vi "Teleop.vi"(10 "Match Info":T4={"Autonomous Elapsed Seconds"=0.0, "TeleOp Elapsed Seconds"=0.0, "Disabled Elapsed Seconds"=0.0, "Visited Autonomous"=FALSE, "Visited TeleOp"=FALSE, "Visited Disabled"=FALSE, "Autonomous Settings"={"Autonomous Style"=enum."Independent", "VI Refnum"=refnum}}, 11 "Call Context":T5) -> ()   [LabVIEW 2018]
doc: "This VI is called for each TeleOp packet received from the DS where the robot is not disabled. It is often used to read from the joysticks and update I/O or to update setpoints for timed control loops. It should complete and return within 20 milliseconds or it may miss DS packets."
uses:
  <vilib>/Rock Robotics/WPI/DriverStation/WPI_DriverStationDerivedRobotMode.ctl
  <vilib>/Rock Robotics/WPI/DriverStation/WPI_DriverStationMatch Info.ctl
  <vilib>/Rock Robotics/WPI/Solenoid/WPI_SolenoidValue.ctl
  <vilib>/Rock Robotics/WPI/ThirdParty/Phoenix-LabVIEW/Motor Controller/Controls/CTRE_Phoenix_MotorControl_ControlMode.ctl
  <vilib>/Rock Robotics/WPI/Utilities/WPI_GetSetVariantRefNum.vi
  <vilib>/Rock Robotics/WPI/Joystick/WPI_JoystickArcadeMapping.vi
  <vilib>/Rock Robotics/Network Tables/NT Write Boolean Array.vi
  <vilib>/Rock Robotics/Network Tables/NT Write Numeric Array.vi
  <vilib>/Rock Robotics/WPI/Solenoid/WPI_SolenoidSetEnum.vi
  <vilib>/Rock Robotics/WPI/ThirdParty/Phoenix-LabVIEW/Motor Controller/Get/CTRE_Phoenix_MotorController_GetSelectedSensorData.vi
  <vilib>/Rock Robotics/Network Tables/NT Read Boolean.vi
  Toolbox/Simple Limit Switch/Limits(Switch+Encoder).vi
  Toolbox/Simple Limit Switch/Limits(DoubleSwitch).vi
  Toolbox/Simple Limit Switch/Limits(SingleSwitch).vi
  <vilib>/Rock Robotics/Network Tables/NT Write Number.vi
panel:
  out "Wrist  Encoder Value":i32
  out "Wrist Out":dbl
  out "Wrist PID Out":dbl
  out "Elevator Out":dbl
  out "Elevator PID Out":dbl
  in  "Outer Invert Motor Limit":bool
  in  "Outer Invert Encoder Limit":bool=TRUE
  in  "Outer Limit":dbl format="%#_13g"
  in  "Horse Invert Encoder Limit":bool=TRUE
  in  "Wrist Invert Encoder Limit":bool=TRUE
  in  "Elevator Invert Encoder Limit":bool=TRUE
  out "Horse Limit Switch":bool
  in  "Reset Horse Encoder":bool
  out "OuterStageSwitch":bool
  out "Wrist After Dangerzone":T1(ring)
  out "Elevator  After Dangerzone":T2(ring)
  in  "Elevator Auto":bool=TRUE
  in  "Elevator Output Range":cluster{"output high":dbl, "output low":dbl}={"output high"=0.2, "output low"=-0.75}
  in  "Elevator PID Gains":T3={"proportional gain (Kc)"=-1e-05, "integral time (Ti, min)"=0.0, "derivative time (Td, min)"=0.0}
  in  "Elevator Setpoints":dbl[](array[numeric])=[-10000.0, -10000.0, -10000.0, 267000.0, 237000.0, 440000.0]
  in  "Wrist Auto":bool=TRUE
  in  "Wrist Output Range":cluster{"output high":dbl, "output low":dbl}={"output high"=0.5, "output low"=-0.5}
  in  "Wrist PID Gains":T3={"proportional gain (Kc)"=2e-05, "integral time (Ti, min)"=0.0, "derivative time (Td, min)"=0.0}
  in  "Wrist Invert Motor Limit":bool=TRUE
  out "Wrist Limit Switch":bool
  out "Elevator Limit Switch Top":bool
  in  "Elevator Invert Motor Limit":bool=TRUE
  in  "Intake Encoder Limit":dbl=-130000.0 format="%#_13g"
  in  "Intake Home Encoder Limit":dbl=-45000.0 format="%#_13g"
  in  "HorseDanger":i32=-600000
  in  "Horse  Encoder Limit":dbl=-190000.0 format="%#_13g"
  in  "Horse Invert Motor Limit":bool=TRUE
  out "Elevator Limit Switch":bool
  out "Elevator Encoder":i32=-47
  in  "Reset Elevator Encoder":bool
  out "Horse Encoder":i32
  in  "Reset Wrist Encoder":bool
  out "Intake Wrist Encoder":i32
  # "BETA POWER/DIRECTIONS\nElevator: Negative is up\nHorse: Negative is into robot\nOuter: Positive is down\nWrist: Negative is into robot"
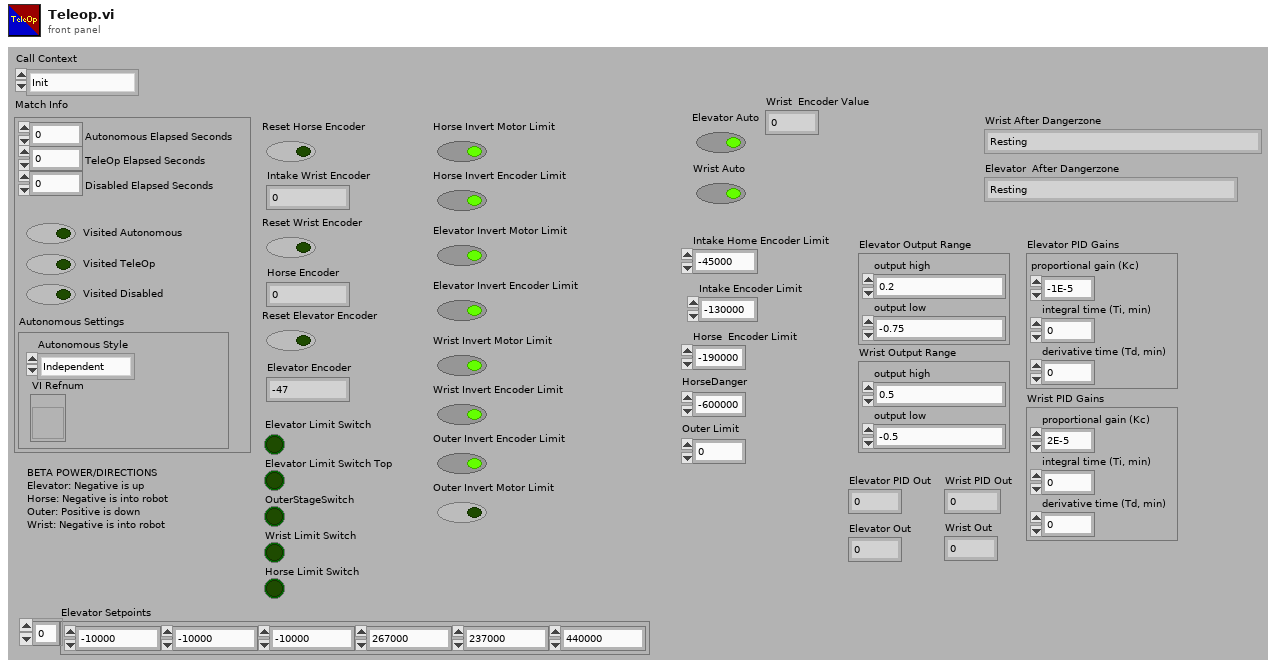
[diagram p1: front panel]
types:
  T1 = enum16{"Resting", "Hatch Ground Intake", "Hatch Place Low/Mid/CargoShip", "Hatch Place High", "Cargo Ground Intake", "Cargo Place Low/Mid", "Cargo Place High", "CargoShip Place Front", "CargoShip Place Back"}
  T2 = enum16{"Resting", "CargoShip Front", "CargoShip Back", "Cargo Mid", "Hatch Mid", "All High"}
  T3 = cluster{"proportional gain (Kc)":dbl, "integral time (Ti, min)":dbl, "derivative time (Td, min)":dbl}
  T4 = typedef "WPI_DriverStationMatch Info.ctl" = cluster{"Autonomous Elapsed Seconds":dbl, "TeleOp Elapsed Seconds":dbl, "Disabled Elapsed Seconds":dbl, "Visited Autonomous":bool, "Visited TeleOp":bool, "Visited Disabled":bool, "Autonomous Settings":cluster{"Autonomous Style":enum16{"Iterative", "Independent"}, "VI Refnum":refnum<vi>}}
  T5 = typedef "WPI_DriverStationDerivedRobotMode.ctl" = enum16{"Init", "Execute", "Stop"}
  T6 = typedef "WPI_SolenoidValue.ctl" = enum16{"Off", "On", "Forward", "Reverse"}
  T7 = enum16{"Intake Cargo", "Outtake Cargo", "Resting Cargo", "Intake Hatches", "Outtake Hatches", "Resting Hatches"}
  T8 = enum16{"Elevator Level 1", "Elevator Level 2", "Elevator Level 3"}
  T9 = typedef "CTRE_Phoenix_MotorControl_ControlMode.ctl" = u16
  T10 = cluster{"Intake Wheels Forwards":bool, "Elevator Shift":bool, "Intake Wheels Backwards":bool, "Drivetrain Shift":bool, "Elevator Outer Forwards":bool, "Elevator Outer Backwards":bool, "Hatch Telescope":bool, "Hatch Intake Clamp":bool, "Horse Drive Up":bool, "Horse Drive Down":bool, "Level 3 Climb":bool}
  T11 = typedef "WPI_JoystickDevRef.ctl" = cluster{"Device":T12}
  T12 = typedef "WPI_JoystickDeviceEnum.ctl" = enum16{"USB 0", "USB 1", "USB 2", "USB 3", "USB 4", "USB 5"}
  T13 = typedef "WPI_MotorControlDeviceRef.ctl" = cluster{"DeviceStatus":errorcluster, "Type":T14, "PWM":cluster{"PWM Channel":T15, "DeadBand":T16}, "CAN":cluster{"Device Number":u8, "SetOutput VI Ref":variant, "GetOutput VI Ref":variant, "Enable VI Ref":variant, "Disable VI Ref":variant, "Data":variant}, "Invert":bool, "DIO PWM":cluster{"PWM \"Enable\" Channel":T15, "DIOChannel":T17, "PWM Rate":dbl}}
  T14 = typedef "WPI_MotorControlType.ctl" = enum16{"PWM", "CAN", "DIO PWM"}
  T15 = typedef "FPGA_DIOPWMChannel.ctl" = enum8{"PWM 0", "PWM 1", "PWM 2", "PWM 3", "PWM 4", "PWM 5", "PWM 6", "PWM 7", "PWM 8", "PWM 9", "PWM MXP 0", "PWM MXP 1", "PWM MXP 2", "PWM MXP 3", "PWM MXP 4", "PWM MXP 5", "PWM MXP 6", "PWM MXP 7", "PWM MXP 8", "PWM MXP 9", "Invalid"}
  T16 = typedef "WPI_PWMDeadband.ctl" = cluster{"Name":string, "maxPositivePwm":i32, "minPositivePwm":i32, "centerPwm":i32, "maxNegativePwm":i32, "minNegativePwm":i32, "angularRange":u16}
  T17 = typedef "FPGA_DIOChannel.ctl" = enum8{"DIO 0", "DIO 1", "DIO 2", "DIO 3", "DIO 4", "DIO 5", "DIO 6", "DIO 7", "DIO 8", "DIO 9", "DIO MXP 0", "DIO MXP 1", "DIO MXP 2", "DIO MXP 3", "DIO MXP 4", "DIO MXP 5", "DIO MXP 6", "DIO MXP 7", "DIO MXP 8", "DIO MXP 9", "DIO MXP 10", "DIO MXP 11", "DIO MXP 12", "DIO MXP 13", "DIO MXP 14", "DIO MXP 15", "SPI Port CS1", "SPI Port CS2", "SPI Port CS3", "SPI Port MISO", "SPI Port MOSI", "Invalid"}
  T18 = typedef "WPI_SolenoidDevRef.ctl" = cluster{"DevStatus":errorcluster, "Pneumatics Control Module":u8, "Forward Solenoid Channel":T19, "Reverse Solenoid Channel":T19}
  T19 = typedef "WPI_SolenoidChannel.ctl" = enum8{"Solenoid 0", "Solenoid 1", "Solenoid 2", "Solenoid 3", "Solenoid 4", "Solenoid 5", "Solenoid 6", "Solenoid 7", "Invalid"}
  T20 = typedef "WPI_SwitchDevRef.ctl" = cluster{"DevStatus":errorcluster, "DIO Channel":T17, "CntIndex":T21, "Normally Closed":bool}
  T21 = typedef "FPGA_CounterCtrSystemIndex.ctl" = enum8{"Ctr 0", "Ctr 1", "Ctr 2", "Ctr 3", "Ctr 4", "Ctr 5", "Ctr 6", "Ctr 7", "Invalid"}
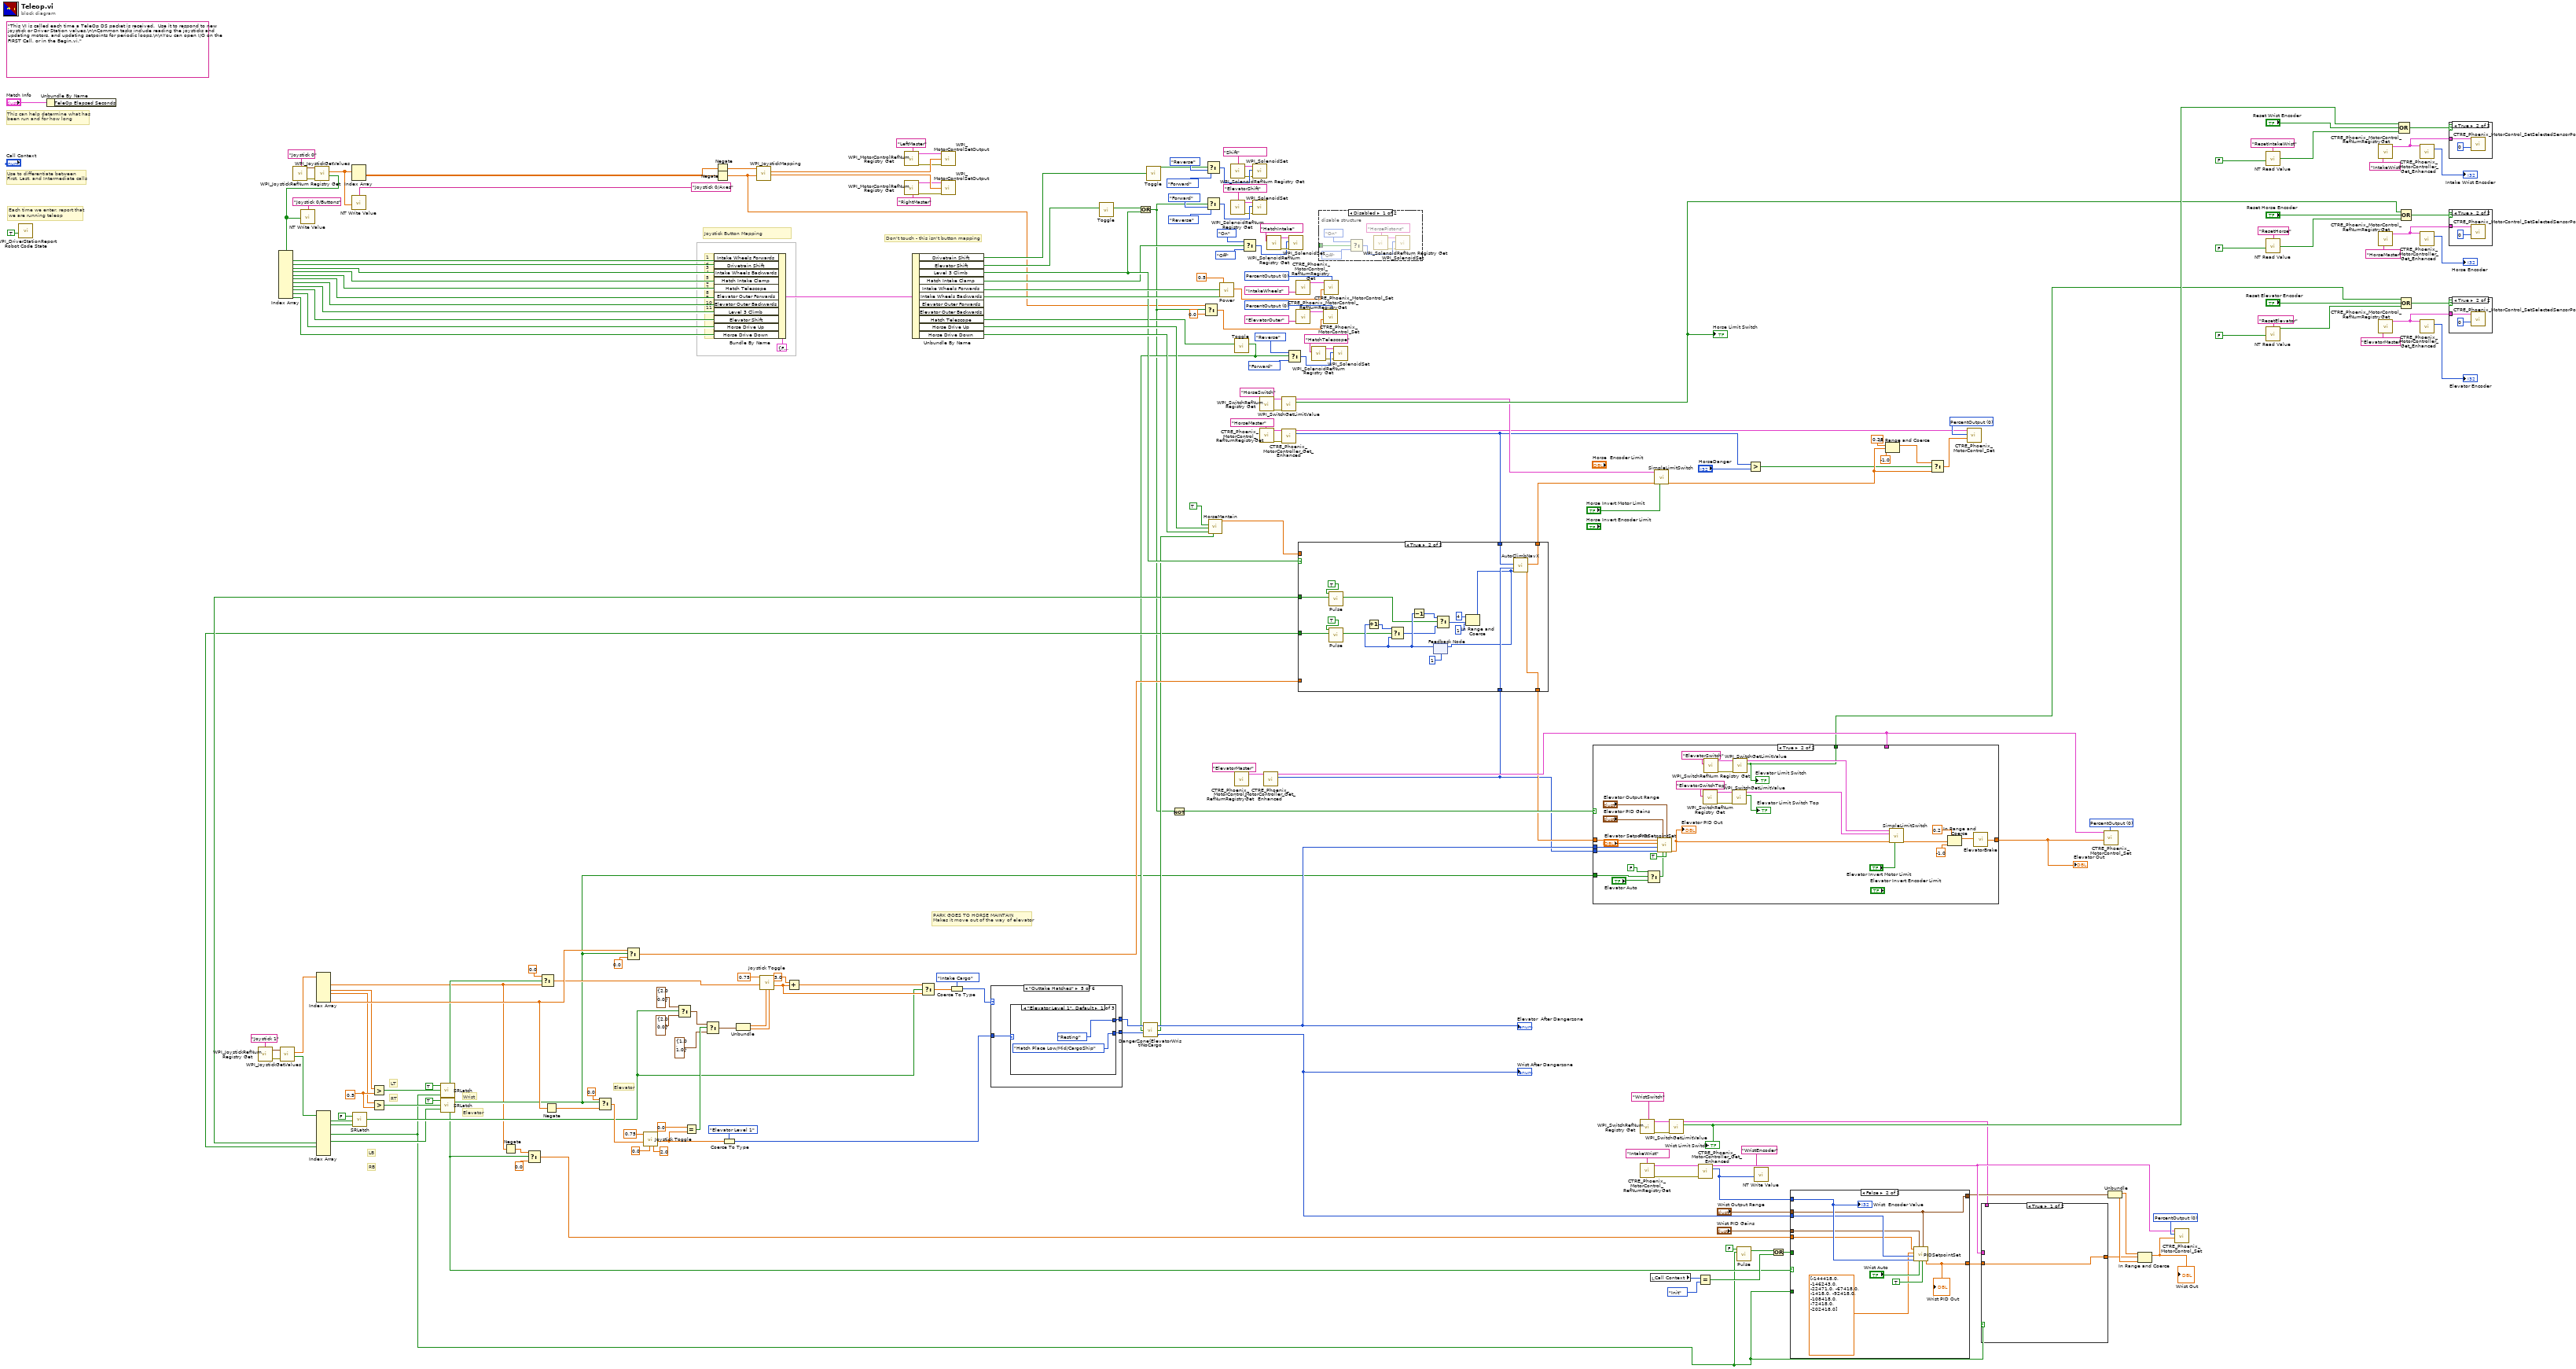
[diagram p0: block diagram]
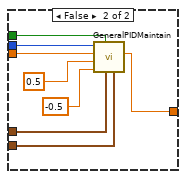
[diagram p3: hidden frame]
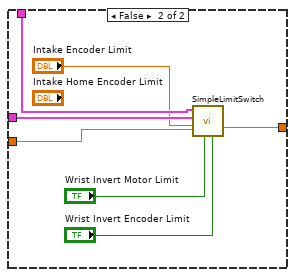
[diagram p4: hidden frame]
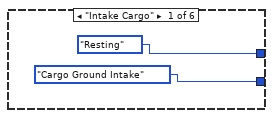
[diagram p6: hidden frame]
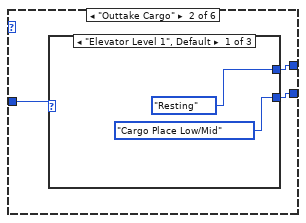
[diagram p7: hidden frame]
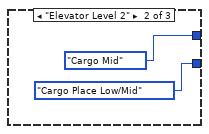
[diagram p8: hidden frame]
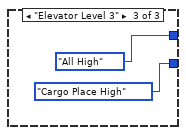
[diagram p9: hidden frame]
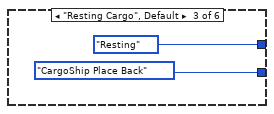
[diagram p10: hidden frame]
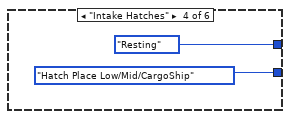
[diagram p11: hidden frame]
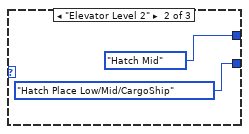
[diagram p12: hidden frame]
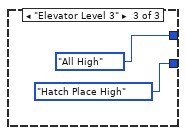
[diagram p13: hidden frame]
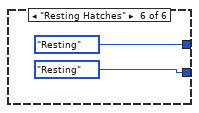
[diagram p14: hidden frame]
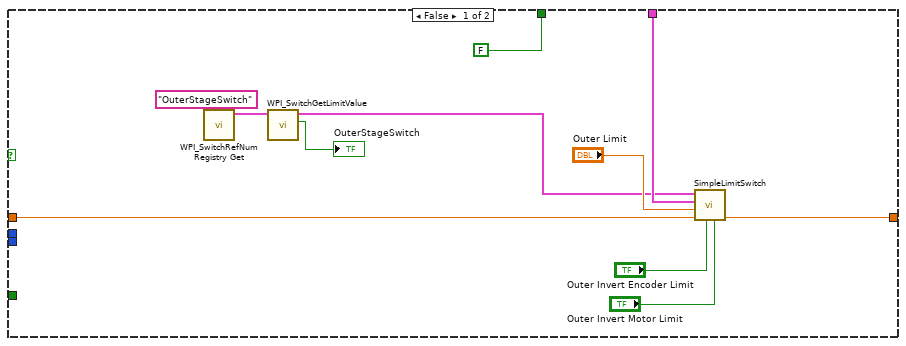
[diagram p16: hidden frame]
diagram:
  w32 = 0.5 ("t")
  w115 = T9 0 items=["PercentOutput"=0, "Position"=1, "Velocity"=2, "Current"=3, "Follower"=5, "MotionProfile"=6, "MotionMagic"=7, "MotionProfileArc"=10, "Disabled"=15] ("Control Mode")
  w119 = T9 0 items=["PercentOutput"=0, "Position"=1, "Velocity"=2, "Current"=3, "Follower"=5, "MotionProfile"=6, "MotionMagic"=7, "MotionProfileArc"=10, "Disabled"=15] ("Control Mode")
  w149 = T9 0 items=["PercentOutput"=0, "Position"=1, "Velocity"=2, "Current"=3, "Follower"=5, "MotionProfile"=6, "MotionMagic"=7, "MotionProfileArc"=10, "Disabled"=15] ("Control Mode")
  w158 = T9 0 items=["PercentOutput"=0, "Position"=1, "Velocity"=2, "Current"=3, "Follower"=5, "MotionProfile"=6, "MotionMagic"=7, "MotionProfileArc"=10, "Disabled"=15] ("Control Mode")
  w160 = T9 0 items=["PercentOutput"=0, "Position"=1, "Velocity"=2, "Current"=3, "Follower"=5, "MotionProfile"=6, "MotionMagic"=7, "MotionProfileArc"=10, "Disabled"=15] ("Control Mode")
  (unwired) "This VI is called each time a TeleOp DS packet is received.  Use it to respond to new joystick or Driver Station values.\n\nCommon tasks include reading the joysticks and updating motors, and updating setpoints for periodic loops.\n\nYou can open I/O on the FIRST Call, or in the Begin.vi."
  # "Elevator"
  # "Elevator"
  # "Wrist"
  # "LT"
  # "RT"
  # "RB"
  # "LB"
  # "Don't touch - this isn't button mapping"
  # "1\n2\n3\n4\n5\n6\n7\n8\n9\n10\n11"
  # "PARK GOES TO HORSE MAINTAIN\nMakes it move out of the way of elevator"
  # "Joystick Button Mapping"
  # "Each time we enter, report that\nwe are running teleop"
  # "Use to differentiate between\nFirst, Last, and Intermediate calls"
  # "This can help determine what has\nbeen run and for how long"
  n1 = call <vilib>:"WPI_DriverStationReport Robot Code State.vi"("TeleOp"=TRUE ("Autonomous")) -> ()  [unwired: 10 in, 1 out]
  n2 = Unbundle By Name("Match Info") -> ()  [unwired: 1 out]
  n3 = call <vilib>:"WPI_JoystickRefNum Registry Get.vi"("refnum name"="Joystick 1") -> ("error out"=w140:errorcluster, "JoystickDevRef"=w139:T11)  [unwired: 9 in]
  n4 = call <vilib>:"WPI_JoystickGetValues.vi"("error in (no error)"=w140, "JoystickDevRef"=w139) -> ("Buttons"=w126:bool[], "Axes"=w127:dbl[])  [unwired: 5 in, 3 out]
  n5 = call <vilib>:"WPI_JoystickRefNum Registry Get.vi"("refnum name"="Joystick 0") -> ("error out"=w188:errorcluster, "JoystickDevRef"=w221:T11)  [unwired: 1 in, 8 out]
  n6 = call <vilib>:"WPI_JoystickGetValues.vi"("error in (no error)"=w188, "JoystickDevRef"=w221) -> ("Buttons"=w185:bool[], "Axes"=w217:dbl[])  [unwired: 5 in, 3 out]
  n7 = Index Array(array=w185) -> (element #1=w205:bool, element #2=w215:bool, element #3=w214:bool, element #4=w213:bool, element #5=w212:bool, element #6=w211:bool, element #7=w210:bool, element #8=w209:bool, element #9=w208:bool, element #10=w207:bool, element #11=w206:bool)  [unwired: 11 in]
  n8 = call-poly <vilib>:"NT Write Value.vi"("Boolean Array"=w185, "Name"="Joystick 0/Buttons") -> ()  [unwired: 9 in, 1 out]
  n9 = Index Array(array=w127) -> (element #2=w7:dbl, element #3=w31:dbl, element #4=w30:dbl, element #6=w68:dbl)  [unwired: 6 in, 2 out]
  n10 = Index Array(array=w126) -> (element #1=w15:bool, element #4=w34:bool, element #5=w4:bool, element #6=w27:bool, element #7=w58:bool, element #8=w57:bool)  [unwired: 10 in, 4 out]
  n11 = Index Array(array=w217) -> (element #1=w164:dbl, element #2=w184:dbl)  [unwired: 2 in]
  n12 = call-poly <vilib>:"NT Write Value.vi"("Numeric Array"=w217, "Name"="Joystick 0/Axes") -> ()  [unwired: 9 in, 1 out]
  n13 = call "SRLatch.vi"("On"=w34, "Off"=w15, "Initial"=FALSE) -> ("Output"=w33:bool)
  n14 = Greater?(x=w31, y=w32) -> (0:w21:bool)
  n15 = Greater?(x=w30, y=w32) -> (0:w20:bool)
  n16 = call "SRLatch.vi"("On"=w4, "Off"=w21, "Initial"=TRUE) -> ("Output"=w9:bool)
  n17 = call "SRLatch.vi"("On"=w27, "Off"=w20, "Initial"=TRUE) -> ("Output"=w8:bool)
  n18 = Negate(x=w7) -> (-x=w70:dbl)
  n19 = Select(t=w70, s=w9, f=0.0) -> (s? t:f=w66:dbl)
  n20 = Select(t=0.0, s=w9, f=w7) -> (s? t:f=w62:dbl)
  n21 = Negate(x=w68) -> (-x=w61:dbl)
  n22 = Select(t=0.0, s=w8, f=w61) -> (s? t:f=w60:dbl)
  n23 = Select(t=w68, s=w8, f=0.0) -> (s? t:f=w67:dbl)
  n24 = call "Joystick Toggle.vi"("Max"=2.0, "Min"=0.0, "Value"=w60, "Range"=0.75) -> ("Output"=w88:dbl)  [unwired: 7 in]
  n25 = Select(t=cluster{"Range":dbl, "Range 2":dbl} {"Range"=2.0, "Range 2"=0.0}, s=w33, f=cluster{"Range":dbl, "Range 2":dbl} {"Range"=2.0, "Range 2"=0.0}) -> (s? t:f=w81:cluster{"Range":dbl, "Range 2":dbl})
  n26 = Equal?(x=0.0, y=w88) -> (x = y?=w80:bool)
  n27 = Select(t=w81, s=w80, f=cluster{"Range":dbl, "Range 2":dbl} {"Range"=1.0, "Range 2"=1.0}) -> (s? t:f=w82:cluster{"Range":dbl, "Range 2":dbl})
  n28 = Bundle By Name(cluster=T10 {"Intake Wheels Forwards"=FALSE, "Elevator Shift"=FALSE, "Intake Wheels Backwards"=FALSE, "Drivetrain Shift"=FALSE, "Elevator Outer Forwards"=FALSE, "Elevator Outer Backwards"=FALSE, "Hatch Telescope"=FALSE, "Hatch Intake Clamp"=FALSE, "Horse Drive Up"=FALSE, "Horse Drive Down"=FALSE, "Level 3 Climb"=FALSE} ("input cluster"), "Intake Wheels Forwards"=w205, "Drivetrain Shift"=w215, "Intake Wheels Backwards"=w214, "Hatch Intake Clamp"=w213, "Hatch Telescope"=w212, "Elevator Outer Forwards"=w211, "Elevator Outer Backwards"=w210, "Level 3 Climb"=w209, "Elevator Shift"=w208, "Horse Drive Up"=w207, "Horse Drive Down"=w206) -> (w204:T10)
  n29 = Negate(x=w164) -> (-x=w25:dbl)
  n30 = Negate(x=w184) -> (-x=w22:dbl)
  n31 = Coerce To Type(0:w88, 1:T8."Elevator Level 1") -> (2:w72:T8)
  n32 = Unbundle(w82) -> ("Range"=w84:dbl, "Range 2"=w83:dbl)
  n33 = call-poly <vilib>:"WPI_JoystickMapping.vi"("Y axis value"=w22, "X axis value"=w25) -> ("Right Motor Value"=w189:dbl, "Left Motor Value"=w190:dbl)  [unwired: 8 in]
  n34 = call "Joystick Toggle.vi"("Max"=w83, "Min"=w84, "Value"=w62, "Range"=0.75) -> ("Output"=w75:dbl)  [unwired: 7 in]
  n35 = Add(x=3.0 ("y"), y=w75) -> (x+y=w76:dbl)
  n36 = call <vilib>:"WPI_MotorControlRefNum Registry Get.vi"("refnum name"="LeftMaster") -> ("error out"=w137:errorcluster, "MotorControlDevRef"=w138:T13)  [unwired: 9 in]
  n37 = call <vilib>:"WPI_MotorControlRefNum Registry Get.vi"("refnum name"="RightMaster") -> ("error out"=w136:errorcluster, "MotorControlDevRef"=w135:T13)  [unwired: 9 in]
  n38 = Unbundle By Name(w204) -> ("Drivetrain Shift"=w183:bool, "Elevator Shift"=w95:bool, "Level 3 Climb"=w94:bool, "Hatch Intake Clamp"=w50:bool, "Intake Wheels Forwards"=w192:bool, "Intake Wheels Backwards"=w191:bool, "Hatch Telescope"=w48:bool, "Horse Drive Up"=w142:bool, "Horse Drive Down"=w143:bool)  [unwired: 2 out]
  n39 = Select(t=w76, s=w33, f=w75) -> (s? t:f=w78:dbl)
  n40 = call <vilib>:"WPI_MotorControlSetOutput.vi"("error in (no error)"=w137, "Output"=w190, "MotorControlDevRef"=w138) -> ()  [unwired: 6 in, 3 out]
  n41 = call <vilib>:"WPI_MotorControlSetOutput.vi"("error in (no error)"=w136, "Output"=w189, "MotorControlDevRef"=w135) -> ()  [unwired: 6 in, 3 out]
  n42 = Coerce To Type(0:w78, 1:T7."Intake Cargo") -> (2:w74:T7)
  n43 = case shown="\"Outtake Hatches\"" w74 {
    tunnel: [T1."Cargo Ground Intake" ("Wrist") w226 T1."CargoShip Place Back" ("Wrist") T1."Hatch Place Low/Mid/CargoShip" ("Wrist") w239 T1."Resting" ("Wrist")] -> w125
    tunnel: [T2."Resting" ("Elevator Level") w227 T2."Resting" ("Elevator Level") T2."Resting" ("Elevator Level") w240 T2."Resting" ("Elevator Level")] -> w123
    tunnel: w72 -> [_ w228 _ _ w241 _]
    frame "Intake Cargo" {
    }
    frame "Outtake Cargo" {
      n44 = case shown="\"Elevator Level 1\", Default" w228 {
        tunnel: [T2."Resting" ("Elevator Level") T2."Cargo Mid" ("Elevator Level") T2."All High" ("Elevator Level")] -> w227
        tunnel: [T1."Cargo Place Low/Mid" ("Wrist") T1."Cargo Place Low/Mid" ("Wrist") T1."Cargo Place High" ("Wrist")] -> w226
        frame "Elevator Level 1", Default {
        }
        frame "Elevator Level 2" {
        }
        frame "Elevator Level 3" {
        }
      }
    }
    frame "Resting Cargo", Default {
    }
    frame "Intake Hatches" {
    }
    frame "Outtake Hatches" {
      n45 = case shown="\"Elevator Level 1\", Default" w241 {
        tunnel: [T2."Resting" ("Elevator Level") T2."Hatch Mid" ("Elevator Level") T2."All High" ("Elevator Level")] -> w240
        tunnel: [T1."Hatch Place Low/Mid/CargoShip" ("Wrist") T1."Hatch Place Low/Mid/CargoShip" ("Wrist") T1."Hatch Place High" ("Wrist")] -> w239
        frame "Elevator Level 1", Default {
        }
        frame "Elevator Level 2" {
        }
        frame "Elevator Level 3" {
        }
      }
    }
    frame "Resting Hatches" {
    }
  }
  n46 = call "Toggle.vi"("Input"=w95) -> ("Output"=w93:bool)  [unwired: 10 in]
  n47 = Or(x=w93, y=w94) -> (x .or. y?=w24:bool)
  n48 = call "Toggle.vi"("Input"=w183) -> ("Output"=w199:bool)  [unwired: 10 in]
  n49 = Not(x=w24) -> (.not. x?=w103:bool)
  n50 = Select(t=w22, s=w24, f=0.0) -> (s? t:f=w26:dbl)
  n51 = Select(t=WPI_SolenoidValue."Reverse" ("Value"), s=w199, f=WPI_SolenoidValue."Forward" ("Value")) -> (s? t:f=w198:T6)
  n52 = Select(t=WPI_SolenoidValue."Forward" ("Value"), s=w24, f=WPI_SolenoidValue."Reverse" ("Value")) -> (s? t:f=w197:T6)
  n53 = call "Power.vi"("Positive Power"=0.5 ("Power"), "Negative"=w191, "Positive"=w192) -> ("Output"=w159:dbl)  [unwired: 8 in]
  n54 = call <vilib>:"WPI_SolenoidRefNum Registry Get.vi"("refnum name"="Shift") -> ("error out"=w186:errorcluster, "SolenoidDevRef"=w202:T18)  [unwired: 9 in]
  n55 = call <vilib>:"WPI_SolenoidRefNum Registry Get.vi"("refnum name"="ElevatorShift") -> ("error out"=w187:errorcluster, "SolenoidDevRef"=w194:T18)  [unwired: 9 in]
  n56 = call "Toggle.vi"("Input"=w48) -> ("Output"=w35:bool)  [unwired: 10 in]
  n57 = call "DangerZone(ElevatorWrist)NoCargo.vi"("Wrist"=w125, "Telescope Out"=w35, "Level"=w123) -> ("Wrist"=w141:T1, "Park Horse"=w64:bool, "Level"=w124:T2)
  "Elevator  After Dangerzone" <- w124
  "Wrist After Dangerzone" <- w141
  n58 = call "HorseMantain.vi"("Park"=w64, "Negative"=w143, "Positive"=w142, "HorseToggle"=TRUE) -> ("Power"=w100:dbl)  [unwired: 7 in]
  n59 = call <vilib>:"CTRE_Phoenix_MotorControl_RefNumRegistryGet.vi"("refnum name"="ElevatorMaster") -> ("PhoenixMotorControlDevRef"=w107:T13)  [unwired: 9 in, 1 out]
  n60 = Select(t=WPI_SolenoidValue."On" ("Value"), s=w50, f=WPI_SolenoidValue."Off" ("Value")) -> (s? t:f=w51:T6)
  n61 = call-poly <vilib>:"WPI_SolenoidSet.vi"("error in (no error)"=w186, "Value"=w198, "SolenoidDevRef"=w202) -> ()  [unwired: 7 in, 2 out]
  n62 = call-poly <vilib>:"WPI_SolenoidSet.vi"("error in (no error)"=w187, "Value"=w197, "SolenoidDevRef"=w194) -> ()  [unwired: 7 in, 2 out]
  n63 = call <vilib>:"WPI_SwitchRefNum Registry Get.vi"("refnum name"="HorseSwitch") -> ("error out"=w122:errorcluster, "SwitchDevRef"=w105:T20)  [unwired: 9 in]
  n64 = call <vilib>:"CTRE_Phoenix_MotorControl_RefNumRegistryGet.vi"("refnum name"="HorseMaster") -> ("error out"=w65:errorcluster, "PhoenixMotorControlDevRef"=w108:T13)  [unwired: 9 in]
  n65 = call-poly <vilib>:"CTRE_Phoenix_MotorController_Get_Enhanced.vi"("PhoenixMotorControlDevRef"=w107) -> ("PhoenixMotorControlDevRef"=w106:T13, "Position (Raw Sensor Units)"=w96:i32)  [unwired: 11 in, 2 out]
  n66 = call <vilib>:"WPI_SolenoidRefNum Registry Get.vi"("refnum name"="HatchIntake") -> ("error out"=w55:errorcluster, "SolenoidDevRef"=w54:T18)  [unwired: 9 in]
  n67 = call <vilib>:"WPI_SwitchGetLimitValue.vi"("error in (no error)"=w122, "SwitchDevRef"=w105) -> ("Switch Pressed"=w132:bool, "SwitchDevRef"=w104:T20)  [unwired: 7 in, 1 out]
  "Horse Limit Switch" <- w132
  n68 = call-poly <vilib>:"CTRE_Phoenix_MotorController_Get_Enhanced.vi"("PhoenixMotorControlDevRef"=w108, "error in"=w65) -> ("PhoenixMotorControlDevRef"=w36:T13, "Position (Raw Sensor Units)"=w101:i32)  [unwired: 10 in, 2 out]
  n69 = Select(t=WPI_SolenoidValue."Reverse" ("Value"), s=w35, f=WPI_SolenoidValue."Forward" ("Value")) -> (s? t:f=w46:T6)
  n70 = call-poly <vilib>:"WPI_SolenoidSet.vi"("error in (no error)"=w55, "Value"=w51, "SolenoidDevRef"=w54) -> ()  [unwired: 7 in, 2 out]
  n71 = call <vilib>:"CTRE_Phoenix_MotorControl_RefNumRegistryGet.vi"("refnum name"="IntakeWheels") -> ("PhoenixMotorControlDevRef"=w161:T13)  [unwired: 9 in, 1 out]
  n72 = call <vilib>:"CTRE_Phoenix_MotorControl_RefNumRegistryGet.vi"("refnum name"="ElevatorOuter") -> ("PhoenixMotorControlDevRef"=w157:T13)  [unwired: 9 in, 1 out]
  n73 = case shown="True" w94 {
    tunnel: w101 -> [_ w270]
    tunnel: [w250 w269] -> w99
    tunnel: [w251 w268] -> w97
    tunnel: w67 -> [w251 _]
    tunnel: w100 -> [w250 _]
    tunnel: w96 -> [_ w267]
    tunnel: w58 -> [_ w257]
    tunnel: w57 -> [_ w254]
    frame False {
    }
    frame True {
      n74 = call "Pulse.vi"("Input"=w257, "Rising Edge?"=TRUE) -> ("Output"=w263:bool)  [unwired: 9 in]
      n75 = call "Pulse.vi"("Input"=w254, "Rising Edge?"=TRUE) -> ("Output"=w260:bool)  [unwired: 9 in]
      n76 = feedback #1(1) -> (w265:i32)
      n77 = Increment(x=w265) -> (x+1=w261:i32)
      n78 = Select(t=w261, s=w260, f=w265) -> (s? t:f=w262:i32)
      n79 = Decrement(x=w265) -> (x-1=w264:i32)
      n80 = Select(t=w264, s=w263, f=w262) -> (s? t:f=w266:i32)
      n81 = In Range and Coerce(upper limit=4, x=w266, lower limit=1) -> (coerced(x)=w252:i32)  [unwired: 1 out]
      n82 = feedback-in #1(w252) -> ()
      n83 = call "AutoClimbNavX.vi"("Stage"=w252, "Elevator Encoder"=w267, "Horse Encoder"=w270) -> ("Elevator Output"=w268:dbl, "Horse Output"=w269:dbl)  [unwired: 7 in]
    }
  }
  n84 = call <vilib>:"WPI_SolenoidRefNum Registry Get.vi"("refnum name"="HatchTelescope") -> ("error out"=w42:errorcluster, "SolenoidDevRef"=w43:T18)  [unwired: 9 in]
  n85 = disable-structure shown="Disabled" {
    disable-tunnel: _ -> [w271 _]
    frame Disabled {
      n86 = Select(t=WPI_SolenoidValue."On" ("Value"), s=w271, f=WPI_SolenoidValue."Off" ("Value")) -> (s? t:f=w277:T6)
      n87 = call <vilib>:"WPI_SolenoidRefNum Registry Get.vi"("refnum name"="HorsePistons") -> ("error out"=w272:errorcluster, "SolenoidDevRef"=w274:T18)  [unwired: 9 in]
      n88 = call-poly <vilib>:"WPI_SolenoidSet.vi"("error in (no error)"=w272, "Value"=w277, "SolenoidDevRef"=w274) -> ()  [unwired: 7 in, 2 out]
    }
    frame Enabled {
    }
  }
  n89 = call <vilib>:"CTRE_Phoenix_MotorControl_Set.vi"("Output"=w26, "Control Mode"=w158, "PhoenixMotorControlDevRef"=w157) -> ()  [unwired: 7 in, 2 out]
  n90 = call <vilib>:"CTRE_Phoenix_MotorControl_Set.vi"("Output"=w159, "Control Mode"=w160, "PhoenixMotorControlDevRef"=w161) -> ()  [unwired: 7 in, 2 out]
  n91 = call-poly <vilib>:"WPI_SolenoidSet.vi"("error in (no error)"=w42, "Value"=w46, "SolenoidDevRef"=w43) -> ()  [unwired: 7 in, 2 out]
  n92 = case shown="True" w103 {
    tunnel: w106 -> [w288 _]
    tunnel: w96 -> [_ w309]
    tunnel: w124 -> [_ w308]
    tunnel: w97 -> [w278 w305]
    tunnel: [w284 w303] -> w102
    tunnel: [FALSE ("Switch Pressed") w294] -> w98
    tunnel: w8 -> [_ w290]
    frame False {
      n93 = call <vilib>:"WPI_SwitchRefNum Registry Get.vi"("refnum name"="OuterStageSwitch") -> ("SwitchDevRef"=w283:T20)  [unwired: 9 in, 1 out]
      n94 = call <vilib>:"WPI_SwitchGetLimitValue.vi"("SwitchDevRef"=w283) -> ("Switch Pressed"=→"OuterStageSwitch":bool, "SwitchDevRef"=w280:T20)  [unwired: 8 in, 1 out]
      n95 = call-poly "SimpleLimitSwitch.vi"("Into Home Limit Is Pos (Encoder)"="Outer Invert Motor Limit", "Into Home Limit Is Pos (Motor)"="Outer Invert Encoder Limit", "Power In"=w278, "Encoder Limit"="Outer Limit", "Motor Ref"=w288, "Limit Switch Ref"=w280) -> ("Power Out"=w284:dbl)  [unwired: 5 in]
    }
    frame True {
      n96 = Select(t=FALSE ("Update"), s=w290, f="Elevator Auto") -> (s? t:f=w291:bool)
      n97 = call "PIDSetpointSet.vi"("Update"=TRUE, "Output Range"="Elevator Output Range", "Auto"=w291, "PID Gains"="Elevator PID Gains", "Encoder Position"=w309, "Level"=w308, "Setpoints"="Elevator Setpoints", "Manual Power"=w305) -> ("Power Out"=w307:dbl)  [unwired: 3 in]
      "Elevator PID Out" <- w307
      n98 = call <vilib>:"WPI_SwitchRefNum Registry Get.vi"("refnum name"="ElevatorSwitchTop") -> ("error out"=w296:errorcluster, "SwitchDevRef"=w298:T20)  [unwired: 9 in]
      n99 = call <vilib>:"WPI_SwitchRefNum Registry Get.vi"("refnum name"="ElevatorSwitch") -> ("error out"=w301:errorcluster, "SwitchDevRef"=w302:T20)  [unwired: 9 in]
      n100 = call <vilib>:"WPI_SwitchGetLimitValue.vi"("error in (no error)"=w296, "SwitchDevRef"=w298) -> ("Switch Pressed"=→"Elevator Limit Switch Top":bool, "SwitchDevRef"=w289:T20)  [unwired: 7 in, 1 out]
      n101 = call <vilib>:"WPI_SwitchGetLimitValue.vi"("error in (no error)"=w301, "SwitchDevRef"=w302) -> ("Switch Pressed"=w294:bool, "SwitchDevRef"=w299:T20)  [unwired: 7 in, 1 out]
      "Elevator Limit Switch" <- w294
      n102 = call-poly "SimpleLimitSwitch.vi"("Into Home Limit Is Pos"="Elevator Invert Motor Limit", "Power In"=w307, "2nd Limit Switch Ref"=w289, "Home Limit Switch Ref"=w299) -> ("Power Out"=w316:dbl)  [unwired: 7 in]
      n103 = In Range and Coerce(upper limit=0.2, x=w316, lower limit=-1.0) -> (coerced(x)=w304:dbl)  [unwired: 1 out]
      n104 = call "ElevatorBrake.vi"("Power In"=w304) -> ("Power Out"=w303:dbl)
    }
  }
  "Elevator Out" <- w102
  n105 = call <vilib>:"WPI_SwitchRefNum Registry Get.vi"("refnum name"="WristSwitch") -> ("error out"=w153:errorcluster, "SwitchDevRef"=w152:T20)  [unwired: 9 in]
  n106 = call <vilib>:"CTRE_Phoenix_MotorControl_RefNumRegistryGet.vi"("refnum name"="IntakeWrist") -> ("error out"=w3:errorcluster, "PhoenixMotorControlDevRef"=w150:T13)  [unwired: 9 in]
  n107 = local read "Call Context"() -> (w14:T5)
  n108 = call-poly "SimpleLimitSwitch.vi"("Into Home Limit Is Pos (Motor)"="Horse Invert Motor Limit", "Power In"=w99, "Limit Switch Ref"=w104) -> ("Power Out"=w111:dbl)  [unwired: 8 in]
  n109 = call <vilib>:"WPI_SwitchGetLimitValue.vi"("error in (no error)"=w153, "SwitchDevRef"=w152) -> ("Switch Pressed"=w144:bool, "SwitchDevRef"=w5:T20)  [unwired: 7 in, 1 out]
  "Wrist Limit Switch" <- w144
  n110 = call-poly <vilib>:"CTRE_Phoenix_MotorController_Get_Enhanced.vi"("PhoenixMotorControlDevRef"=w150, "error in"=w3) -> ("PhoenixMotorControlDevRef"=w148:T13, "Position (Raw Sensor Units)"=w2:i32)  [unwired: 10 in, 2 out]
  n111 = Equal?(x=w14, y=WPI_DriverStationDerivedRobotMode."Init") -> (x = y?=w10:bool)
  n112 = call "Pulse.vi"("Input"=w4, "Rising Edge?"=FALSE) -> ("Output"=w12:bool)  [unwired: 9 in]
  n113 = Greater?(x=w101, y="HorseDanger") -> (0:w109:bool)
  n114 = call-poly <vilib>:"NT Write Value.vi"("Numeric"=w2, "Name"="WristEncoder") -> ()  [unwired: 9 in, 1 out]
  n115 = Or(x=w12, y=w10) -> (x .or. y?=w11:bool)
  n116 = case shown="False" w9 {
    tunnel: w2 -> [w321 w341]
    tunnel: w141 -> [_ w340]
    tunnel: [w322 w339] -> w128
    tunnel: w66 -> [w323 w337]
    tunnel: [w319 w334] -> w40
    tunnel: "Wrist PID Gains" -> [w320 w335]
    tunnel: "Wrist Output Range" -> [w319 w334]
    tunnel: w4 -> [w318 _]
    tunnel: w11 -> [w317 _]
    frame True {
      n117 = case shown="True" w318 {
        tunnel: w323 -> [w324 w332]
        tunnel: [w324 w331] -> w322
        tunnel: w321 -> [_ w330]
        tunnel: w320 -> [_ w327]
        tunnel: w319 -> [_ w326]
        tunnel: w317 -> [_ w325]
        frame True {
        }
        frame False {
          n118 = call "GeneralPIDMaintain.vi"("PID gains"=w327, "Output Range"=w326, "Initialize"=w325, "Lower Power Limit"=-0.5, "Upper Power Limit"=0.5, "Power"=w332, "Encoder Position"=w330) -> ("Power Out"=w331:dbl)  [unwired: 4 in]
        }
      }
    }
    frame False {
      n119 = call "PIDSetpointSet.vi"("Update"=TRUE, "Output Range"=w334, "Auto"="Wrist Auto", "PID Gains"=w335, "Encoder Position"=w341, "Level"=w340, "Setpoints"=dbl[] [-144418.0, -146243.0, -22471.0, -67418.0, -1418.0, -92418.0, -108418.0, -72418.0, -202418.0] ("Wrist Setpoints"), "Manual Power"=w337) -> ("Power Out"=w339:dbl)  [unwired: 3 in]
      "Wrist PID Out" <- w339
      "Wrist  Encoder Value" <- w341
    }
  }
  n120 = In Range and Coerce(upper limit=0.25, x=w111, lower limit=-1.0) -> (coerced(x)=w112:dbl)  [unwired: 1 out]
  n121 = Select(t=w112, s=w109, f=w111) -> (s? t:f=w110:dbl)
  n122 = call <vilib>:"CTRE_Phoenix_MotorControl_Set.vi"("Output"=w110, "Control Mode"=w119, "PhoenixMotorControlDevRef"=w36) -> ()  [unwired: 7 in, 2 out]
  n123 = case shown="True" w4 {
    tunnel: [w342 w349] -> w37
    tunnel: w148 -> [_ w348]
    tunnel: w128 -> [w342 w345]
    tunnel: w5 -> [_ w344]
    frame True {
    }
    frame False {
      n124 = call-poly "SimpleLimitSwitch.vi"("Into Home Limit Is Pos (Encoder)"="Wrist Invert Encoder Limit", "Into Home Limit Is Pos (Motor)"="Wrist Invert Motor Limit", "Power In"=w345, "Encoder Limit"="Intake Encoder Limit", "Motor Ref"=w348, "Limit Switch Ref"=w344) -> ("Power Out"=w349:dbl)  [unwired: 5 in]
    }
  }
  n125 = call <vilib>:"CTRE_Phoenix_MotorControl_Set.vi"("Output"=w102, "Control Mode"=w115, "PhoenixMotorControlDevRef"=w106) -> ()  [unwired: 7 in, 2 out]
  n126 = Unbundle(w40) -> ("output high"=w39:dbl, "output low"=w38:dbl)
  n127 = In Range and Coerce(upper limit=w39, x=w37, lower limit=w38) -> (coerced(x)=w41:dbl)  [unwired: 1 out]
  "Wrist Out" <- w41
  n128 = call <vilib>:"CTRE_Phoenix_MotorControl_Set.vi"("Output"=w41, "Control Mode"=w149, "PhoenixMotorControlDevRef"=w148) -> ()  [unwired: 7 in, 2 out]
  n129 = call-poly <vilib>:"NT Read Value.vi"("Default Value"=FALSE, "Name"="ResetIntakeWrist") -> ("Boolean"=w172:bool)  [unwired: 8 in, 1 out]
  n130 = call-poly <vilib>:"NT Read Value.vi"("Default Value"=FALSE, "Name"="ResetHorse") -> ("Boolean"=w169:bool)  [unwired: 8 in, 1 out]
  n131 = call-poly <vilib>:"NT Read Value.vi"("Default Value"=FALSE, "Name"="ResetElevator") -> ("Boolean"=w147:bool)  [unwired: 8 in, 1 out]
  n132 = call <vilib>:"CTRE_Phoenix_MotorControl_RefNumRegistryGet.vi"("refnum name"="IntakeWrist") -> ("PhoenixMotorControlDevRef"=w180:T13)  [unwired: 9 in, 1 out]
  n133 = call <vilib>:"CTRE_Phoenix_MotorControl_RefNumRegistryGet.vi"("refnum name"="HorseMaster") -> ("PhoenixMotorControlDevRef"=w179:T13)  [unwired: 9 in, 1 out]
  n134 = call <vilib>:"CTRE_Phoenix_MotorControl_RefNumRegistryGet.vi"("refnum name"="ElevatorMaster") -> ("PhoenixMotorControlDevRef"=w174:T13)  [unwired: 9 in, 1 out]
  n135 = Compound Arithmetic op=OR(w144, "Reset Wrist Encoder", w172) -> (w129:bool)
  n136 = Compound Arithmetic op=OR(w132, "Reset Horse Encoder", w169) -> (w130:bool)
  n137 = Compound Arithmetic op=OR(w98, "Reset Elevator Encoder", w147) -> (w131:bool)
  n138 = call-poly <vilib>:"CTRE_Phoenix_MotorController_Get_Enhanced.vi"("PhoenixMotorControlDevRef"=w180) -> ("Position (Raw Sensor Units)"=→"Intake Wrist Encoder":i32)  [unwired: 11 in, 3 out]
  n139 = call-poly <vilib>:"CTRE_Phoenix_MotorController_Get_Enhanced.vi"("PhoenixMotorControlDevRef"=w179) -> ("Position (Raw Sensor Units)"=→"Horse Encoder":i32)  [unwired: 11 in, 3 out]
  n140 = call-poly <vilib>:"CTRE_Phoenix_MotorController_Get_Enhanced.vi"("PhoenixMotorControlDevRef"=w174) -> ("Position (Raw Sensor Units)"=→"Elevator Encoder":i32)  [unwired: 11 in, 3 out]
  n141 = case shown="True" w129 {
    tunnel: w180 -> [_ w351]
    frame False {
    }
    frame True {
      n142 = call <vilib>:"CTRE_Phoenix_MotorControl_SetSelectedSensorPosition.vi"("New Sensor Position"=0, "PhoenixMotorControlDevRef"=w351) -> ()  [unwired: 8 in, 2 out]
    }
  }
  n143 = case shown="True" w130 {
    tunnel: w179 -> [_ w353]
    frame False {
    }
    frame True {
      n144 = call <vilib>:"CTRE_Phoenix_MotorControl_SetSelectedSensorPosition.vi"("New Sensor Position"=0, "PhoenixMotorControlDevRef"=w353) -> ()  [unwired: 8 in, 2 out]
    }
  }
  n145 = case shown="True" w131 {
    tunnel: w174 -> [_ w355]
    frame False {
    }
    frame True {
      n146 = call <vilib>:"CTRE_Phoenix_MotorControl_SetSelectedSensorPosition.vi"("New Sensor Position"=0, "PhoenixMotorControlDevRef"=w355) -> ()  [unwired: 8 in, 2 out]
    }
  }
